vi "Begin.vi"(8 "error in (no error)":errorcluster, 9 "Left":T1, 10 "Right":T1, 11 "Drive in":refnum<class "Drive.lvclass">) -> (0 "error out":errorcluster, 3 "Drive out":refnum<class "Drive.lvclass">)   [LabVIEW 2018, in "Drive.lvlib" / "Drive.lvclass"]
doc: "This VI holds the begin code"
uses:
  Drive.lvclass
  Pod Drive/Pod.ctl
  Pod Drive/Pod Drive.lvclass
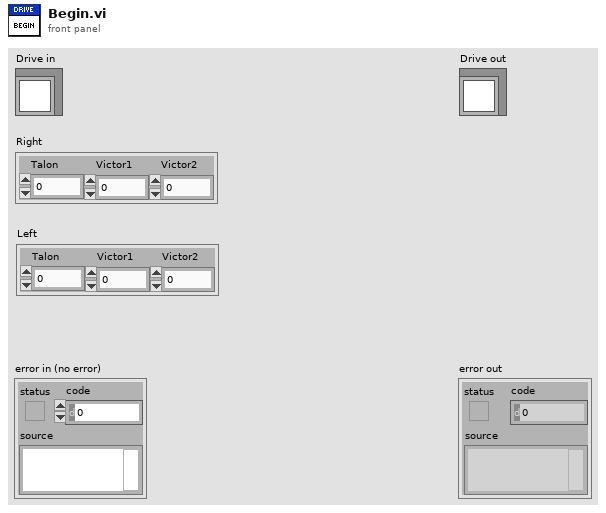
[diagram p1: front panel]
types:
  T1 = typedef "Drive.lvlib/Pod Drive.lvclass/Pod.ctl" = cluster{"Talon":u8, "Victor1":u8, "Victor2":u8}
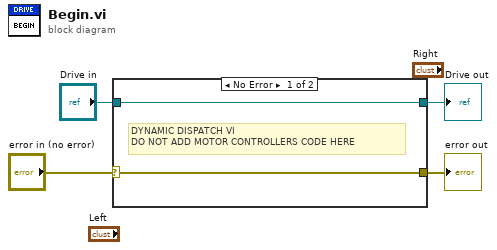
[diagram p0: block diagram]
diagram:
  n1 = case shown="No Error" "error in (no error)" {
    selector: "error in (no error)" -> [w5 w8]
    tunnel: [w5 w8] -> w3
    tunnel: [w6 w7] -> w1
    tunnel: "Drive in" -> [w6 w7]
    frame No Error {
      # "DYNAMIC DISPATCH VI\nDO NOT ADD MOTOR CONTROLLERS CODE HERE"
    }
    frame Error {
    }
  }
  "error out" <- w3
  "Drive out" <- w1
